vi "Main.vi"() -> ()   [LabVIEW 2013]
uses:
  state.ctl
panel:
  out "function":bool
  out "display":string
  in  "ESC":bool
  out "stack":i32[](array[numeric])
  # "RPN Calculator"
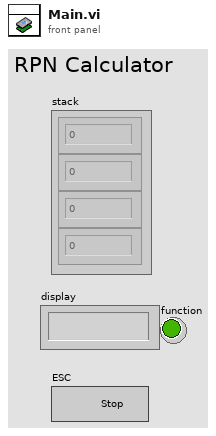
[diagram p1: front panel]
types:
  T1 = typedef "state.ctl" = enum16{"idle", "digit", "enter", "clear", "add", "change sign", "multiply", "function", "square", "square root"}
  T2 = typedef "keypad references.ctl" = cluster{"column drivers":T3, "row drivers":T3, "pull downs":bool, "timeout [ms]":u32}
  T3 = typedef "DIO.lvlib/DIO Reference.ctl" = cluster{"myRIO Reference":T4, "DIO Channels List":T8}
  T4 = typedef "myRIO Generic Hardware Reference.ctl" = cluster{"myRIO Model":T5, "myRIO Hardware Reference":T6}
  T5 = typedef "Hardware Version Enum.ctl" = enum16{"Unknown", "myRIO-1900", "myRIO-1950"}
  T6 = typedef "myRIO v1.0 Reference.ctl" = cluster{"Generic FPGA Reference":T7, "Allow multiple opens":bool}
  T7 = typedef "Generic FPGA Reference.ctl" = refnum<k20>
  T8 = typedef "DIO Channels List.ctl" = T9[]
  T9 = typedef "DIO Channels Enum.ctl" = enum16{"Not Connected", "C/DIO0", "C/DIO1", "C/DIO2", "C/DIO3", "C/DIO4", "C/DIO5", "C/DIO6", "C/DIO7", "A/DIO0", "A/DIO1", "A/DIO2", "A/DIO3", "A/DIO4", "A/DIO5", "A/DIO6", "A/DIO7", "A/DIO8", "A/DIO9", "A/DIO10", "A/DIO11", "A/DIO12", "A/DIO13", "A/DIO14", "A/DIO15", "B/DIO0", "B/DIO1", "B/DIO2", "B/DIO3", "B/DIO4", "B/DIO5", "B/DIO6", "B/DIO7", "B/DIO8", "B/DIO9", "B/DIO10", "B/DIO11", "B/DIO12", "B/DIO13", "B/DIO14", "B/DIO15", "LED0", "LED1", "LED2", "LED3", "Button0"}
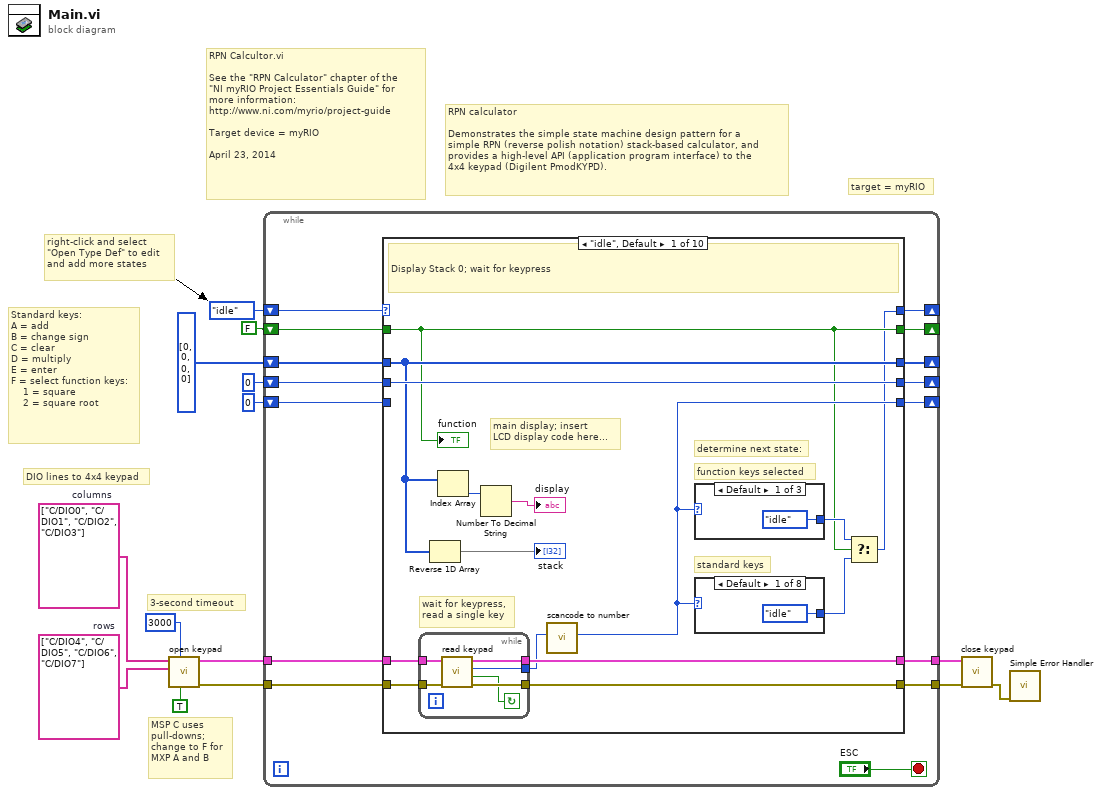
[diagram p0: block diagram]
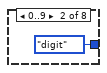
[diagram p2: hidden frame]
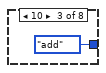
[diagram p3: hidden frame]
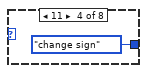
[diagram p4: hidden frame]
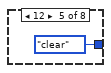
[diagram p5: hidden frame]
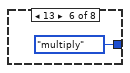
[diagram p6: hidden frame]
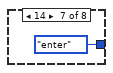
[diagram p7: hidden frame]
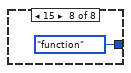
[diagram p8: hidden frame]
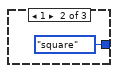
[diagram p9: hidden frame]
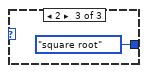
[diagram p10: hidden frame]
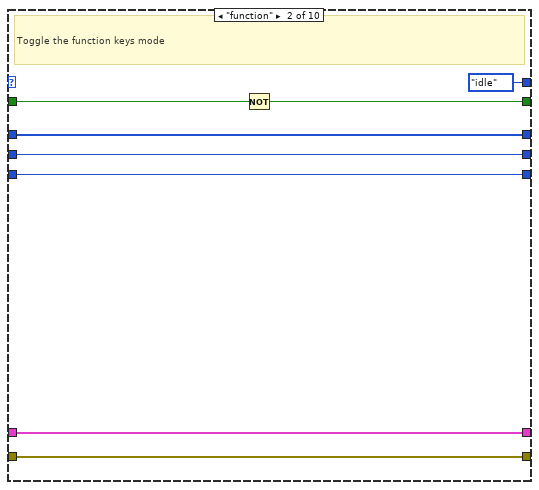
[diagram p11: hidden frame]
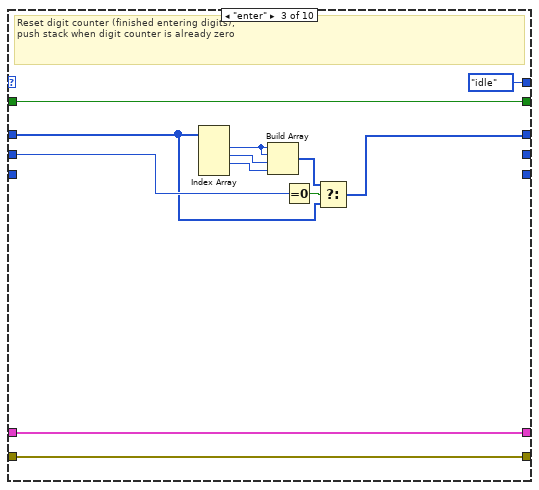
[diagram p12: hidden frame]
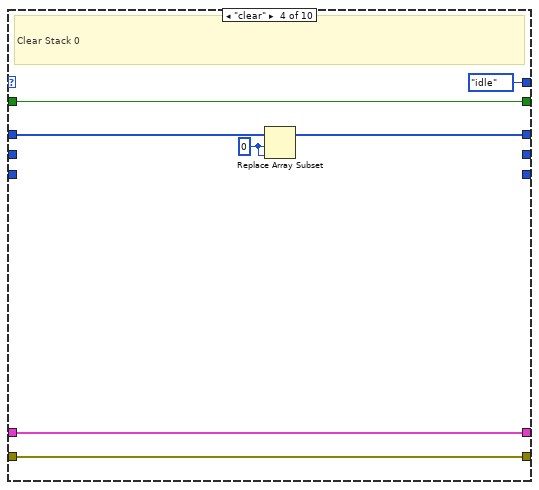
[diagram p13: hidden frame]
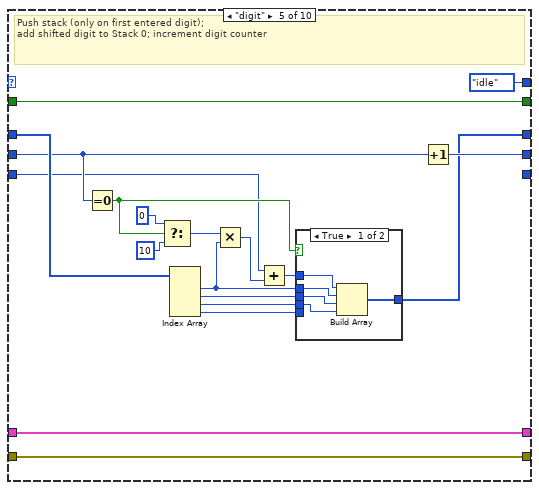
[diagram p14: hidden frame]
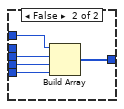
[diagram p15: hidden frame]
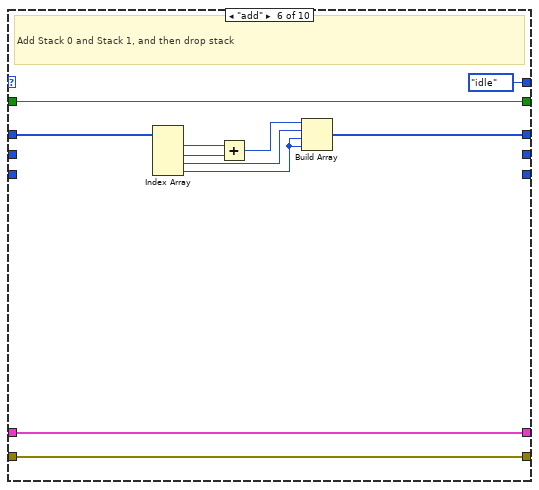
[diagram p16: hidden frame]
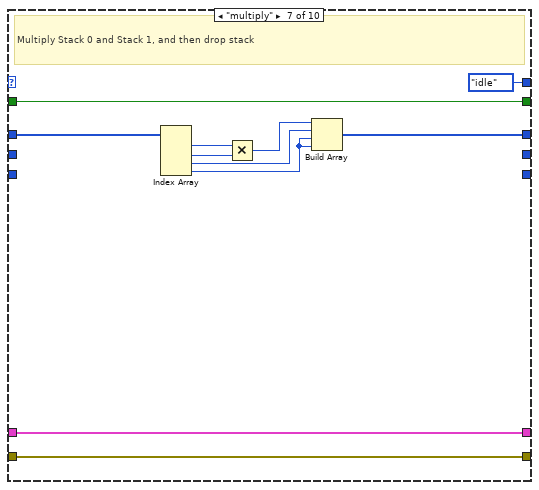
[diagram p17: hidden frame]
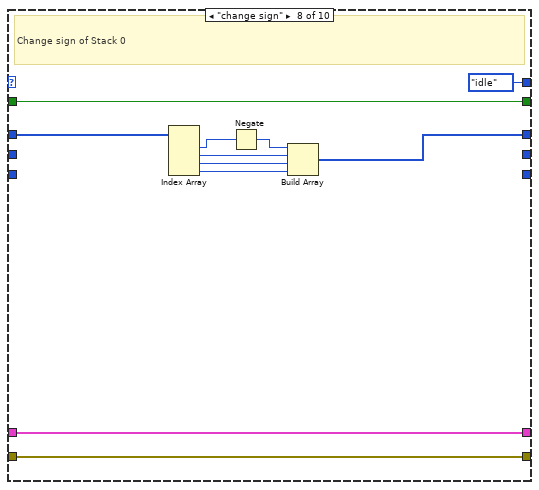
[diagram p18: hidden frame]
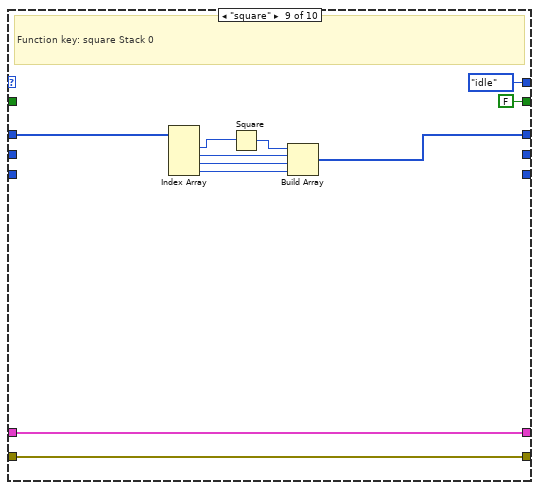
[diagram p19: hidden frame]
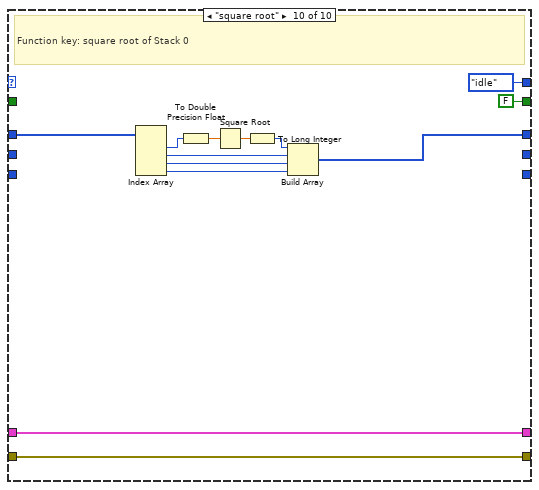
[diagram p20: hidden frame]
diagram:
  w11 = tag[] ["C/DIO4", "C/DIO5", "C/DIO6", "C/DIO7"]  # rows
  w12 = tag[] ["C/DIO0", "C/DIO1", "C/DIO2", "C/DIO3"]  # columns
  # "RPN Calcultor.vi\n\nSee the \"RPN Calculator\" chapter of the \n\"NI myRIO Project Essentials Guide\" for\nmore information: \nhttp://www.ni.com/myrio/project-guide\n\nTarget device = myRIO\n\nApril 23, 2014"
  # "Standard keys:\nA = add\nB = change sign\nC = clear\nD = multiply\nE = enter\nF = select function keys:\n    1 = square\n    2 = square root"
  # "target = myRIO"
  # "RPN calculator\n\nDemonstrates the simple state machine design pattern for a\nsimple RPN (reverse polish notation) stack-based calculator, and\nprovides a high-level API (application program interface) to the\n4x4 keypad (Digilent PmodKYPD)."
  # "right-click and select\n\"Open Type Def\" to edit\nand add more states"
  # "3-second timeout"
  # "MSP C uses\npull-downs;\nchange to F for\nMXP A and B"
  # "DIO lines to 4x4 keypad"
  n1 = call "open keypad.vi"("pull downs"=TRUE, "timeout [ms]"=u32 3000, "rows"=w11, "columns"=w12) -> ("error out"=w7:errorcluster, "keypad ref out"=w8:T2)  [unwired: 6 in]
  n2 = while {
    shift-right: [w29] -> _
    shift-left: state."idle" ("state") -> [w28]
    shift-right: [w22] -> _
    shift-left: i32[] [0, 0, 0, 0] -> [w27]
    tunnel: w8 -> [w26]
    tunnel: w7 -> [w25]
    tunnel: [w24] -> w6
    tunnel: [w23] -> w5
    shift-right: [w20] -> _
    shift-left: 0 -> [w21]
    shift-right: [w19] -> _
    shift-left: 0 ("keypad value") -> [w18]
    shift-right: [w16] -> _
    shift-left: FALSE ("pull downs") -> [w15]
    stop <- "ESC" stop-if-true
    n3 = case shown="\"idle\", Default" w28 {
      tunnel: [w30 state."idle" ("state") state."idle" ("state") state."idle" ("state") state."idle" ("state") state."idle" ("state") state."idle" ("state") state."idle" ("state") state."idle" ("state") state."idle" ("state")] -> w29
      tunnel: w27 -> [w36 w69 w71 w88 w105 w128 w134 w150 w161 w174]
      tunnel: w26 -> [w44 w66 w80 w84 w102 w119 w131 w142 w153 w168]
      tunnel: w25 -> [w43 w65 w79 w83 w101 w120 w130 w141 w152 w167]
      tunnel: [w42 w65 w79 w83 w101 w120 w130 w141 w152 w167] -> w24
      tunnel: [w41 w66 w80 w84 w102 w119 w131 w142 w153 w168] -> w23
      tunnel: [w36 w69 w72 w86 w103 w124 w133 w144 w155 w170] -> w22
      tunnel: w21 -> [w39 w68 w78 _ w100 _ _ _ _ _]
      tunnel: [w39 w68 _ _ w106 _ _ _ _ _] -> w20
      tunnel: [w34 w67 _ _ _ _ _ _ _ _] -> w19
      tunnel: w18 -> [_ w67 _ _ w89 _ _ _ _ _]
      tunnel: [w31 w63 w77 w82 w91 w118 w129 w140 FALSE ("pull downs") FALSE ("pull downs")] -> w16
      tunnel: w15 -> [w31 w64 w77 w82 w91 w118 w129 w140 _ _]
      frame "idle", Default {
        # "determine next state:"
        # "main display; insert\nLCD display code here..."
        # "wait for keypress,\nread a single key"
        # "standard keys"
        # "function keys selected"
        # "Display Stack 0; wait for keypress"
        n4 = while {
          tunnel: w44 -> [w58]
          tunnel: w43 -> [w57]
          tunnel: [w56] -> w42
          tunnel: [w55] -> w41
          tunnel: [w54] -> w40
          stop <- w53 continue-if-true
          n5 = call "read keypad.vi"("error in (no error)"=w57, "keypad ref"=w58) -> ("error out"=w56:errorcluster, "timed out"=w53:bool, "keypad code"=w54:i32, "keypad ref out"=w55:T2)  [unwired: 6 in]
        }
        n6 = Reverse 1D Array(array=w36) -> (reversed array=→"stack":i32[])
        n7 = Index Array "Index Array"(array=w36) -> (element=w38:i32)  [unwired: 1 in]
        n8 = Number To Decimal String(number=w38) -> (decimal integer string=→"display":string)  [unwired: 1 in]
        n9 = call "scancode to number.vi"("keypad code"=w40) -> ("keypad value"=w34:i32)  [unwired: 10 in]
        n10 = case shown="Default" w34 {
          tunnel: [state."idle" ("state") state."square" ("state") state."square root" ("state")] -> w33
          frame Default {
          }
          frame 1 {
          }
          frame 2 {
          }
        }
        n11 = case shown="Default" w34 {
          tunnel: [state."idle" ("state") state."digit" ("state") state."add" ("state") state."change sign" ("state") state."clear" ("state") state."multiply" ("state") state."enter" ("state") state."function" ("state")] -> w32
          frame Default {
          }
          frame 0..9 {
          }
          frame 10 {
          }
          frame 11 {
          }
          frame 12 {
          }
          frame 13 {
          }
          frame 14 {
          }
          frame 15 {
          }
        }
        n12 = Select(t=w33, s=w31, f=w32) -> (s? t:f=w30:T1)
        "function" <- w31
      }
      frame "function" {
        # "Toggle the function keys mode"
        n13 = Not(x=w64) -> (.not. x?=w63:bool)
      }
      frame "enter" {
        # "Reset digit counter (finished entering digits);\npush stack when digit counter is already zero"
        n14 = Index Array "Index Array"(array=w71) -> (element #1=w76:i32, element #2=w75:i32, element #3=w74:i32)  [unwired: 4 in, 1 out]
        n15 = Build Array "Build Array"(w76, w76, w75, w74) -> (w73:i32[])
        n16 = Equal To 0?(x=w78) -> (x = 0?=w70:bool)
        n17 = Select(t=w73, s=w70, f=w71) -> (s? t:f=w72:i32[])
      }
      frame "clear" {
        w87 = 0 ("index")
        # "Clear Stack 0"
        n18 = Replace Array Subset "Replace Array Subset"(array=w88, new element=w87, index=w87) -> (w86:i32[])
      }
      frame "digit" {
        # "Push stack (only on first entered digit); \nadd shifted digit to Stack 0; increment digit counter"
        n19 = Equal To 0?(x=w100) -> (x = 0?=w96:bool)
        n20 = Select(t=0, s=w96, f=10) -> (s? t:f=w92:i32)
        n21 = Index Array "Index Array"(array=w105) -> (element #1=w93:i32, element #2=w97:i32, element #3=w98:i32, element #4=w99:i32)  [unwired: 4 in]
        n22 = Multiply(x=w92, y=w93) -> (x*y=w90:i32)
        n23 = Add(x=w89, y=w90) -> (x+y=w104:i32)
        n24 = case shown="True" w96 {
          tunnel: w104 -> [w111 w117]
          tunnel: [w112 w116] -> w103
          tunnel: w93 -> [w110 _]
          tunnel: w99 -> [_ w115]
          tunnel: w98 -> [w108 w114]
          tunnel: w97 -> [w109 w113]
          frame True {
            n25 = Build Array "Build Array"(w111, w110, w109, w108) -> (w112:i32[])
          }
          frame False {
            n26 = Build Array "Build Array"(w117, w113, w114, w115) -> (w116:i32[])
          }
        }
        n27 = Increment(x=w100) -> (x+1=w106:i32)
      }
      frame "add" {
        # "Add Stack 0 and Stack 1, and then drop stack"
        n28 = Index Array "Index Array"(array=w128) -> (element #1=w126:i32, element #2=w127:i32, element #3=w123:i32, element #4=w122:i32)  [unwired: 4 in]
        n29 = Add(x=w126, y=w127) -> (x+y=w125:i32)
        n30 = Build Array "Build Array"(w125, w123, w122, w122) -> (w124:i32[])
      }
      frame "multiply" {
        # "Multiply Stack 0 and Stack 1, and then drop stack"
        n31 = Index Array "Index Array"(array=w134) -> (element #1=w138:i32, element #2=w139:i32, element #3=w136:i32, element #4=w135:i32)  [unwired: 4 in]
        n32 = Multiply(x=w138, y=w139) -> (x*y=w137:i32)
        n33 = Build Array "Build Array"(w137, w136, w135, w135) -> (w133:i32[])
      }
      frame "change sign" {
        # "Change sign of Stack 0"
        n34 = Index Array "Index Array"(array=w150) -> (element #1=w149:i32, element #2=w147:i32, element #3=w146:i32, element #4=w145:i32)  [unwired: 4 in]
        n35 = Negate(x=w149) -> (-x=w148:i32)
        n36 = Build Array "Build Array"(w148, w147, w146, w145) -> (w144:i32[])
      }
      frame "square" {
        # "Function key: square Stack 0"
        n37 = Index Array "Index Array"(array=w161) -> (element #1=w160:i32, element #2=w158:i32, element #3=w157:i32, element #4=w156:i32)  [unwired: 4 in]
        n38 = Square(x=w160) -> (x^2=w159:i32)
        n39 = Build Array "Build Array"(w159, w158, w157, w156) -> (w155:i32[])
      }
      frame "square root" {
        # "Function key: square root of Stack 0"
        n40 = Index Array "Index Array"(array=w174) -> (element #1=w164:i32, element #2=w173:i32, element #3=w172:i32, element #4=w171:i32)  [unwired: 4 in]
        n41 = To Double Precision Float(number=w164) -> (double precision float=w166:dbl)
        n42 = Square Root(x=w166) -> (sqrt(x)=w165:dbl)
        n43 = To Long Integer(number=w165) -> (32bit integer=w163:i32)
        n44 = Build Array "Build Array"(w163, w173, w172, w171) -> (w170:i32[])
      }
    }
  }
  n45 = call "close keypad.vi"("error in (no error)"=w6, "keypad ref out"=w5) -> ("error out"=w1:errorcluster)  [unwired: 9 in]
  n46 = call <vilib>:"Simple Error Handler.vi"("error in (no error)"=w1) -> ()  [unwired: 4 in, 5 out]
